vi "Read.vi"(0 "reference in":refnum<class "Torque.lvclass">, 5 "error in (no error)":errorcluster) -> (14 "reference out":refnum<class "Torque.lvclass">, 19 "error out":errorcluster)   [LabVIEW 2013, in "Torque.lvclass"]
uses:
  Torque.lvclass
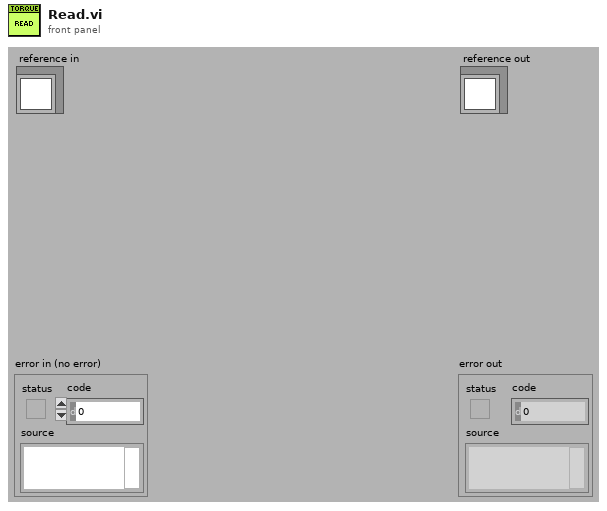
[diagram p1: front panel]
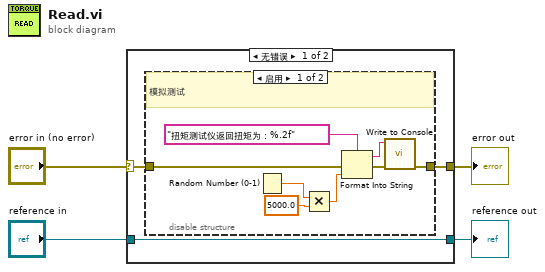
[diagram p0: block diagram]
diagram:
  n1 = case shown="无错误" "error in (no error)" {
    selector: "error in (no error)" -> [w6 w18]
    tunnel: [w5 w18] -> w3
    tunnel: [w7 w17] -> w1
    tunnel: "reference in" -> [w7 w17]
    frame No Error {
      n2 = disable-structure shown="启用" {
        disable-tunnel: w6 -> [w10 w16]
        disable-tunnel: [w15 w16] -> w5
        frame Enabled {
          # "模拟测试"
          n3 = Random Number (0-1)() -> (number: 0 to 1=w14:dbl)
          n4 = Multiply(x=w14, y=5000.0) -> (x*y=w12:dbl)
          n5 = Format Into String(format string="扭矩测试仪返回扭矩为：%.2f" ("Input"), error in=w10, w12) -> (resulting string=w8:string, error out=w9:errorcluster)  [unwired: 1 in]
          n6 = call "Write to Console.vi"("error in (no error)"=w9, "Input"=w8) -> ("error out"=w15:errorcluster)  [unwired: 9 in]
        }
        frame Disabled {
          # "实际测试"
        }
      }
    }
    frame Error {
    }
  }
  "error out" <- w3
  "reference out" <- w1
